vi "Scope1.vi"(2 "错误输入":errorcluster caption="错误输出") -> (0 "错误输出":errorcluster)   [LabVIEW 2018]
uses:
  <instrlib>/Tektronix DPO MSO 2000 4000 Series/Public/Configure/Configure Trigger (Edge).vi
  InOut/Reslut.vi
  <instrlib>/Tektronix DPO MSO 2000 4000 Series/Tektronix DPO MSO 2000 4000 Series.lvlib
panel:
  in  "结果输出":i32(listbox)
  in  "衰减挡位":T1 scale=1.0..4.0
  in  "触发电压":u64(ring)=200 items=["200mv"=200, "200mv"=0, "100mv"=100, "20mv"=20, "10mv"=10, "2mv"=2, "1mv"=1]
  in  "输入阻抗/Ω":u64(ring)=2 items=["1M", "75", "50"]
  out "时间波形":waveform(dbl)(graph)
  in  "电压范围":u64(ring)=10 items=["5v/dim"=5000000, "1v/dim"=1000000, "500mv/dim"=500000, "100mv/dim"=100000, "50mv/dim"=50000, "10mv/dim"=10000, "5mv/dim"=5000, "1mv/dim"=1000, "500uv/dim"=500, "100uv/dim"=100, "50uv/dim"=50, "10uv/dim"=10]
  in  "时间范围":u64(ring)=100000 items=["100ms/dim"=1000000000, "50ms/dim"=500000000, "10ms/dim"=100000000, "5ms/dim"=50000000, "1ms/dim"=10000000, "500us/dim"=5000000, "100us/dim"=1000000, "50us/dim"=500000, "10us/dim"=100000, "5us/dim"=50000, "1us/dim"=10000, "500ns/dim"=5000, "100ns/dim"=1000, "50ns/dim"=500, "10ns/dim"=100, "5ns/dim"=50, "1ns/dim"=10, "500ps/dim"=5, "100ps/dim"=1]
  in  "Channel":T2(ring)
  in  "测量状态":enum16{"设置参数", "等待", "采集", "结束", "调整衰减"}(ring)
  out "重频":string
  out "脉宽":string
  in  "结束测量":bool
  # "时间波形"
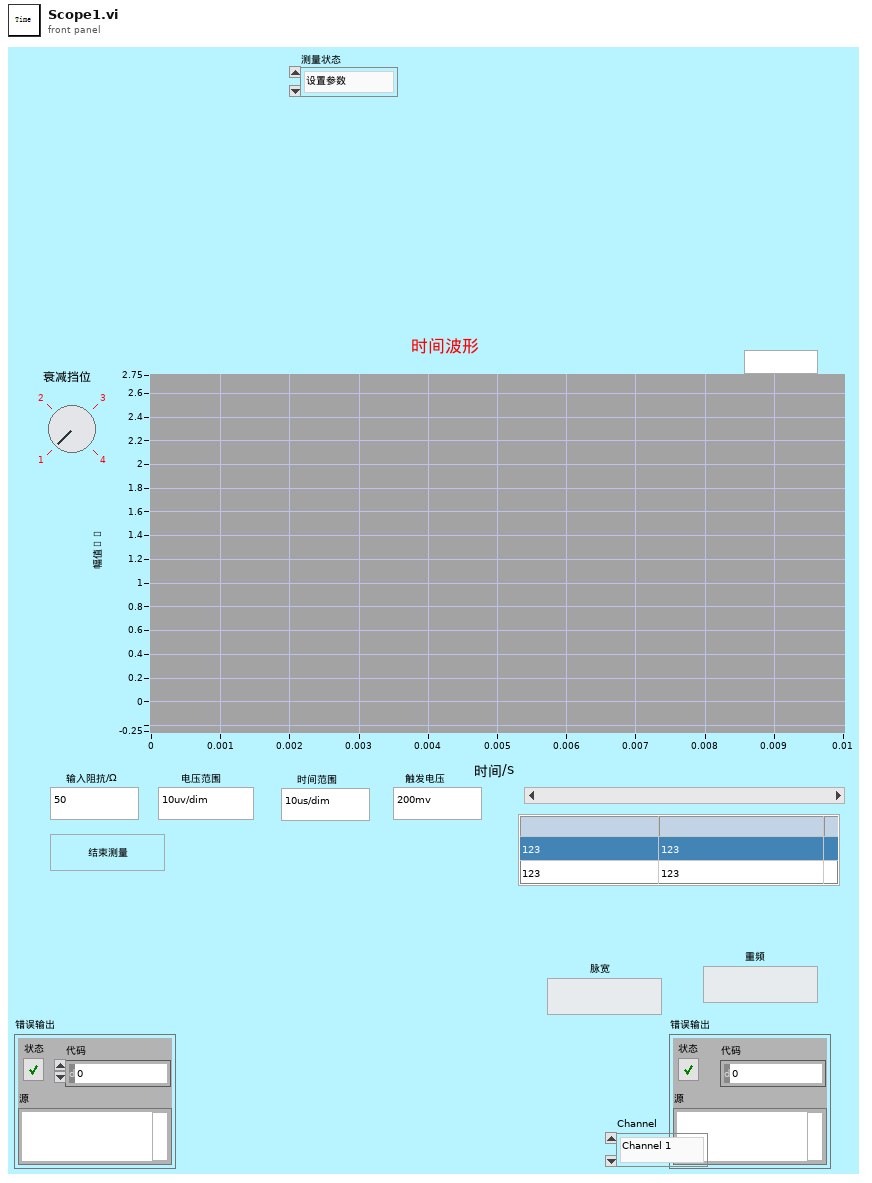
[diagram p1: front panel]
types:
  T1 = typedef "衰减片前面板.ctl" = u8
  T2 = enum16{"Channel 1", "Channel 2", "Channel 3", "Channel 4"}
  T3 = enum16{"光谱测量", "功率测量", "能量测量", "时间波形", "偏振测量", "近远场"}
  T4 = typedef "衰减片电机指令枚举器.ctl" = enum16{"归0", "停止", "运动", "轴设置", "通信连接", "读取位置"}
  T5 = typedef "衰减片电机枚举.ctl" = enum16{"小积分球衰减", "偏振仪衰减", "近场相机衰减", "远场相机衰减"}
  T6 = enum8{"Enabled", "Disabled", "Disabled and Grayed Out"}
  T7 = typedef "控制电机位置枚举器.ctl" = enum16{"远场扫描", "发散角扫描", "远场相机", "近场相机", "时间波形", "偏振", "能量", "功率", "光谱"}
  T8 = typedef "控制电机指令枚举器.ctl" = enum16{"归0", "停止", "运动", "轴设置", "通信连接"}
  T9 = typedef "控制电机枚举器.ctl" = enum16{"Z", "Y", "X", "发散角", "俯仰", "旋转"}
  T10 = enum16{"光谱测量", "功率测量", "能量测量", "时间波形测量", "偏振测量", "近远场测量"}
  T11 = typedef "衰减片电机位置枚举器.ctl" = enum16{"0倍", "10倍", "100倍", "1000倍"}
  T12 = cluster{"激光器型号":string, "X":dbl, "Y":dbl, "Z":dbl, "Rotate":dbl, "Pitching":dbl, "DivergeAngle":dbl, "衰减片位置":cluster{"小积分球位置":T11, "偏振仪位置 ":T11, "近场相机位置 ":T11, "远场相机位置":T11}, "Type":string, "Serial":string}
  T13 = typedef "IMAQ Image.ctl" = refnum<image>
  T14 = cluster{"示波器":cluster{"Channel (0:Channel 1)":enum16{"Channel 1", "Channel 2", "Channel 3", "Channel 4"}, "电压范围":dbl, "触发电压":dbl, "时间范围":dbl, " 示波器VISA":refnum<visa-resource-name>, "时间范围 标签":u64, "电压范围 标签":u64, "触发电压 标签":u64, "输入阻抗/Ω":u64, "示波器类型":bool}, "光谱仪":cluster{"SpecDataReference":refnum<queue>, "grating center":dbl, "Exposure Time (s)":dbl, "是否进行详细设置":bool, " 开始通信检查":bool, "通信成功？":bool, "波长":dbl, "LightField Automation out":refnum<class "LightField Automation.lvclass">}, " 近场相机":cluster{"曝光时间/us":dbl, "IP 地址":string, "ImageData":T13, " 曝光最大":i32, " 曝光最小":i32, "Camera Source":refnum<k21>, "近场X范围":dbl, "近场Y范围":dbl, "单个像元大小/um":dbl, "相机距离原点位置":dbl[], "是否测量发散角":bool, "光束类型(发散T)":bool, "聚焦透镜焦距mm":dbl}, " 偏振仪":cluster{"电压范围":u64, "触发电压":u64, "时间范围":u64, "波长范围":enum16{"可见光 400-700nm", "近红外 700-1100nm"}, "可见光偏振测量仪VISA":refnum<visa-resource-name>, "近红外偏振测量仪VISA":refnum<visa-resource-name>}, " 功率计":cluster{"通道":enum16{"Channel 1", "Channel 2"}, "工作波长":u32, "单位":u64, "时间范围":u64, "IP地址":string, "端口":u32, "是否需要散射片":bool}, "能量计":cluster{"通道":enum16{"Channel 1", "Channel 2"}, "工作波长":u32, "单位":u64, "时间范围":u64, "IP地址":string, "端口":u32, "能量计量程":enum16{"200uJ", "20uJ", "2uJ", "200nJ"}}, "电机":cluster{"Channel (0:Channel 1)":enum16{"Channel 1", "Channel 2", "Channel 3", "Channel 4"}, "电压范围":u64, "触发电压":u64, "时间范围":u64}, " 远场相机":cluster{"曝光时间/us":i32, "IP 地址":string, "ImageData":T13, "  增益最大":i32, "  增益最小":i32, " 曝光最大":i32, " 曝光最小":i32, "ImageData B":T13, "是否远场测量":bool}}
  T15 = cluster{"Channel (0:Channel 1)":enum16{"Channel 1", "Channel 2", "Channel 3", "Channel 4"}, "电压范围":dbl, "触发电压":dbl, "时间范围":dbl, " 示波器VISA":refnum<visa-resource-name>, "时间范围 标签":u64, "电压范围 标签":u64, "触发电压 标签":u64, "输入阻抗/Ω":u64, "示波器类型":bool}
  T16 = cluster{"波形":waveform(dbl), "脉宽":string, "重频":string, "脉冲宽度Uint":string, "重复频率Uint":string}
  T17 = cluster{"任务":cluster{"功率任务":bool, "能量任务":bool, "时间波形任务":bool, "光谱任务":bool, "偏振任务":bool, "近远场任务":bool}, "通信":cluster{"功率通信":bool, "能量通信":bool, "时间波形通信":bool, "光谱通信":bool, "偏振通信":bool, "近远场通信":bool}}
  T18 = cluster{"功率通信":bool, "能量通信":bool, "时间波形通信":bool, "光谱通信":bool, "偏振通信":bool, "近远场通信":bool}
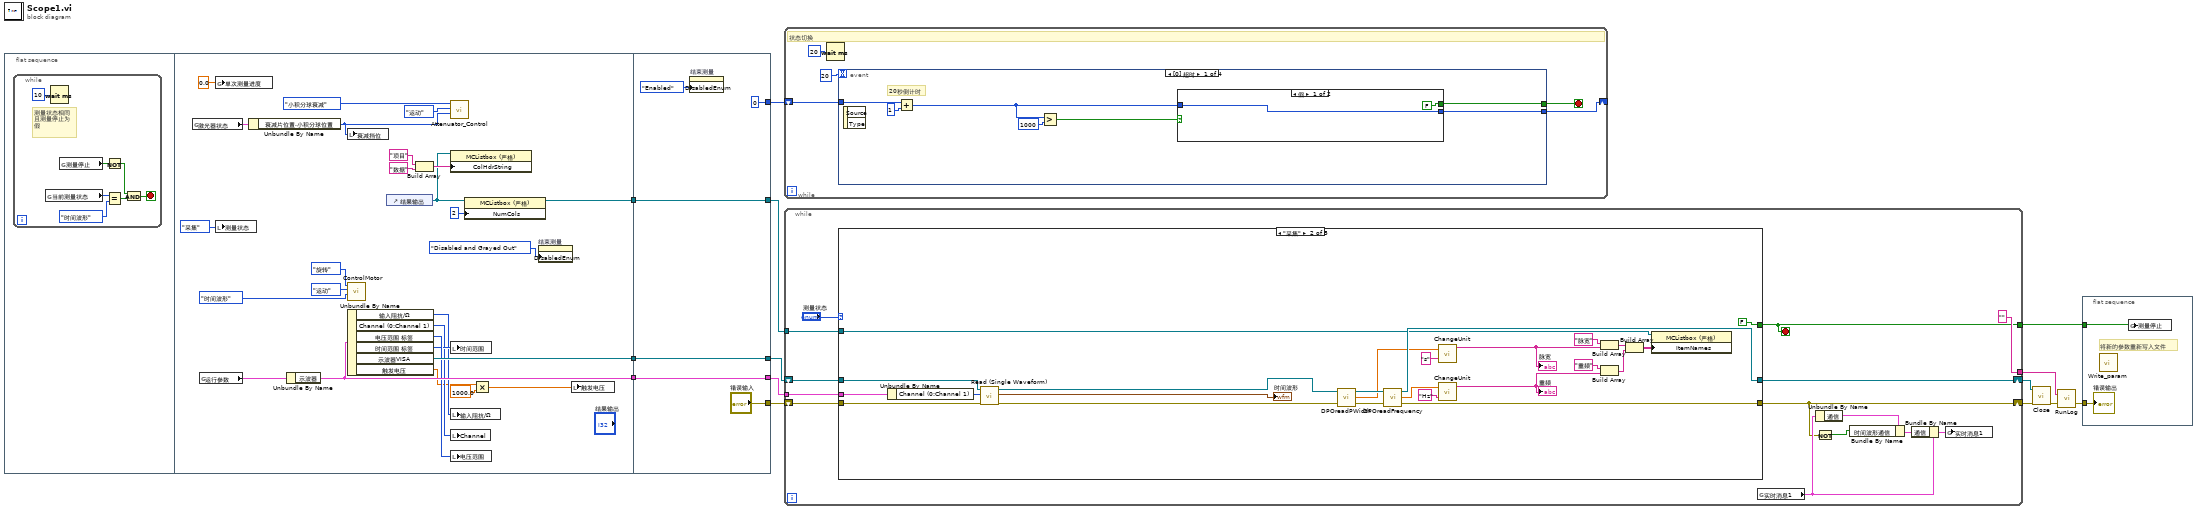
[diagram p0: block diagram]
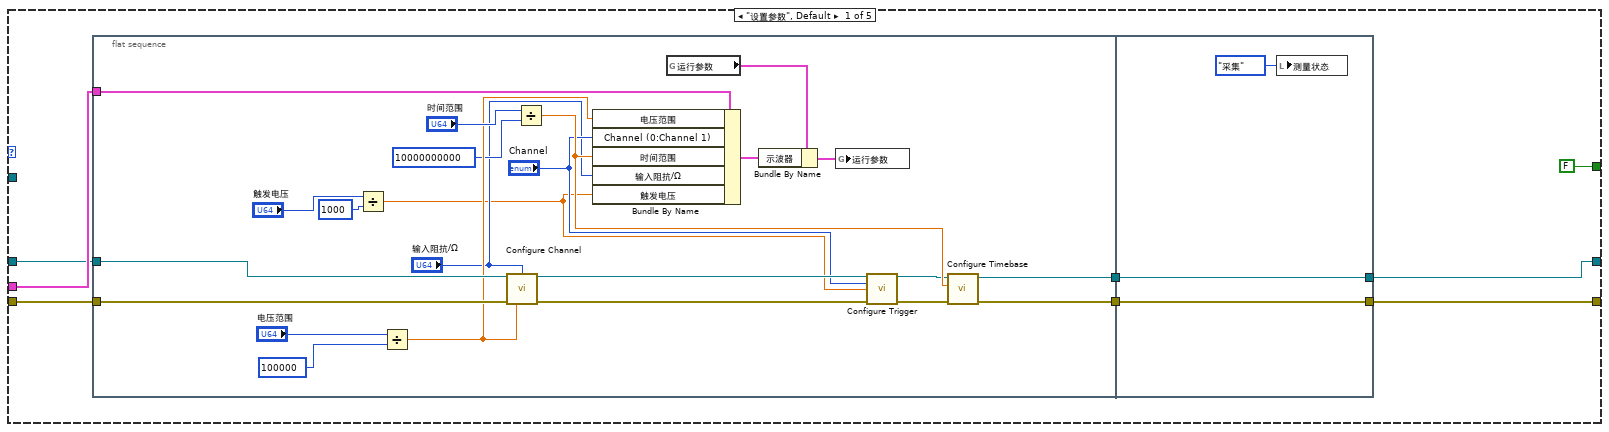
[diagram p2: hidden frame]
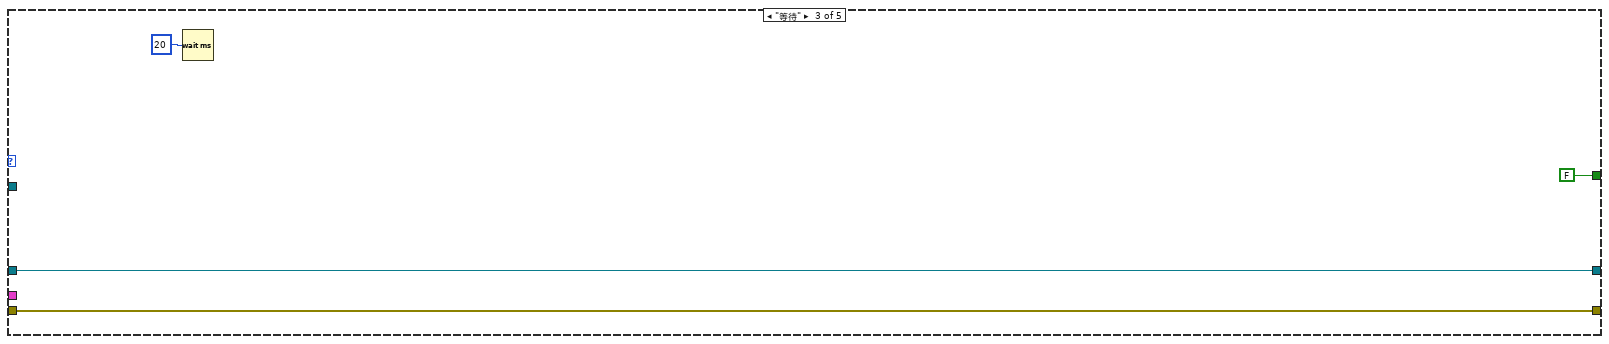
[diagram p3: hidden frame]
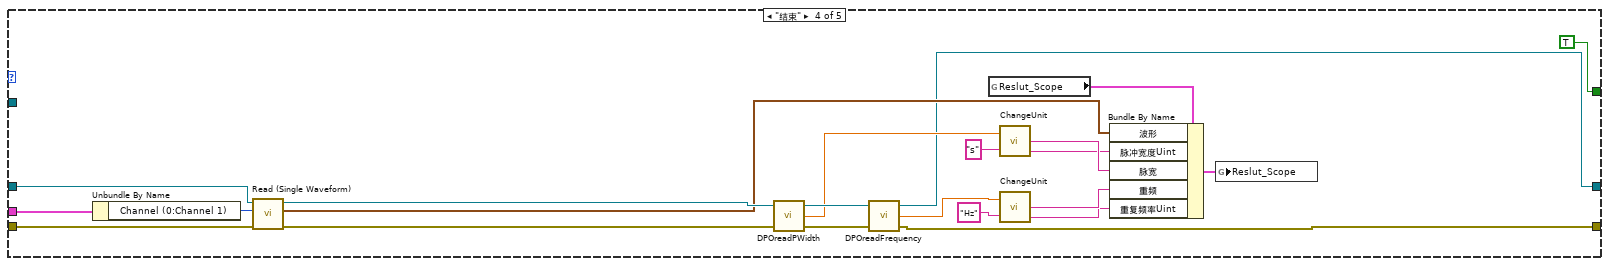
[diagram p4: hidden frame]
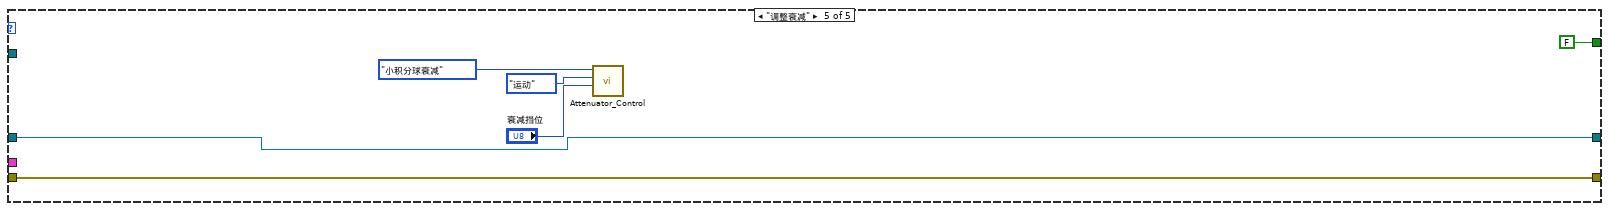
[diagram p5: hidden frame]
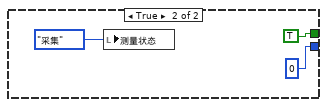
[diagram p6: hidden frame]
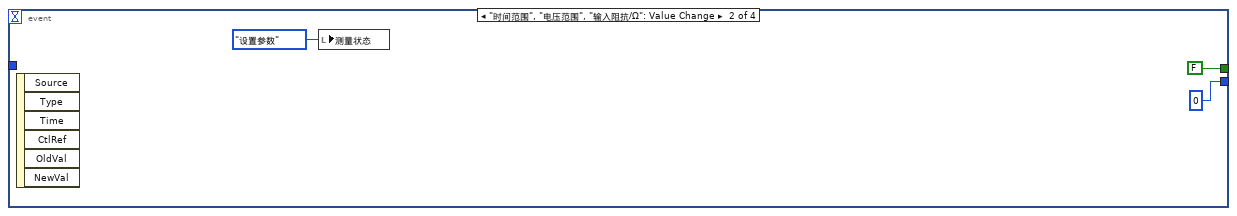
[diagram p7: hidden frame]
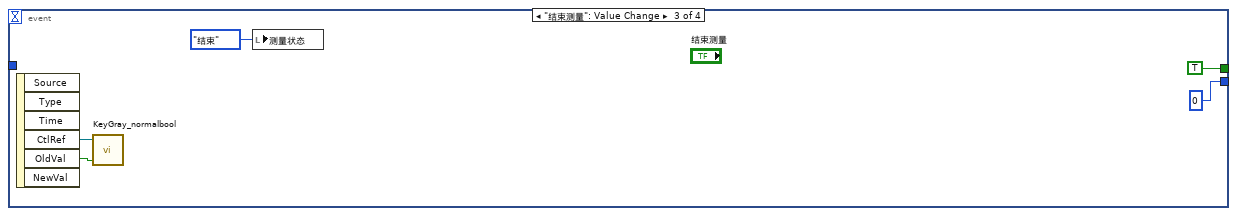
[diagram p8: hidden frame]
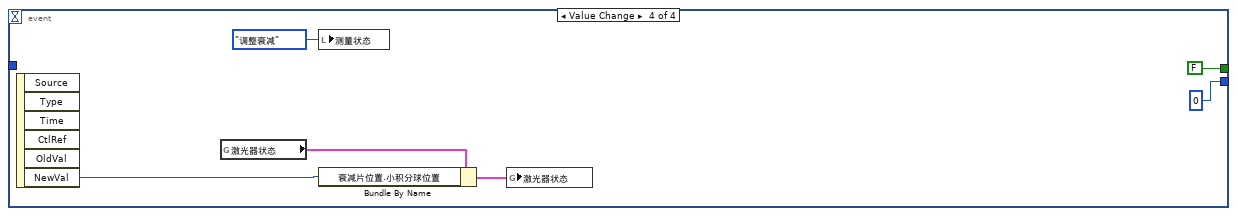
[diagram p9: hidden frame]
diagram:
  n1 = flat-sequence {
    tunnel: [w47] -> w6
    tunnel: [w45] -> w5
    tunnel: [w22] -> w2
    tunnel: [w52] -> w13
    tunnel: [w53] -> w14
    tunnel: w6 -> [w53]
    tunnel: w5 -> [w52]
    tunnel: [0] -> w7
    tunnel: [w49] -> w3
    tunnel: w2 -> [w49]
    tunnel: ["错误输入"] -> w1
    frame #0 {
      n2 = while {
        stop <- w19 stop-if-true
        # "测量状态相同\n且测量停止为\n假"
        n3 = global read "参数.vi" "当前测量状态"() -> (w21:T10)
        n4 = Wait (ms)(milliseconds to wait=u32 10 ("等待时间（毫秒）")) -> ()  [unwired: 1 out]
        n5 = global read "参数.vi" "测量停止"() -> (w17:bool)
        n6 = Not(x=w17) -> (.not. x?=w18:bool)
        n7 = Equal?(x=w21, y=T3."时间波形" ("当前测量状态")) -> (x = y?=w16:bool)
        n8 = And(x=w18, y=w16) -> (x .and. y?=w19:bool)
      }
    }
    frame #1 {
      n9 = global read "参数.vi" "激光器状态"() -> (w35:T12)
      n10 = global read "参数.vi" "运行参数"() -> (w46:T14)
      n11 = global write "globalMessage.vi" "单次测量进度"(0.0 ("单次测量进度")) -> ()
      n12 = local write "测量状态"(enum16{"设置参数", "等待", "采集"}."采集" ("测量状态")) -> ()
      n13 = Unbundle By Name(w35) -> ("衰减片位置.小积分球位置"=w28:T11)
      n14 = Unbundle By Name(w46) -> ("示波器"=w45:T15)
      n15 = local write "衰减挡位"(w28) -> ()
      n16 = call "ControlMotor.vi"("控制电机"=控制电机枚举器."旋转", "控制电机指令"=控制电机指令枚举器."运动", "位置"=控制电机位置枚举器."时间波形") -> ()  [unwired: 5 in, 1 out]
      n17 = Unbundle By Name(w45) -> ("输入阻抗/Ω"=w40:u64, "Channel (0:Channel 1)"=w41:T2, "电压范围 标签"=w44:u64, "时间范围 标签"=w43:u64, "示波器VISA"=w47:refnum<visa-resource-name>, "触发电压"=w39:dbl)
      n18 = control-ref of="结果输出"() -> (w23:refnum<vi>)
      n19 = Build Array("项目", "数据") -> (w24:string[])
      n20 = call "Attenuator_Control.vi"("位置"=w28, "控制电机指令"=衰减片电机指令枚举器."运动", "电机"=衰减片电机枚举."小积分球衰减") -> ()  [unwired: 2 in, 2 out]
      n21 = property on="属性节点" class="MCListbox (严格)"(reference=w23, "ColHdrString"=w24) -> ()  [unwired: 1 in, 2 out]
      n22 = local write "时间范围"(w43) -> ()
      n23 = local write "输入阻抗/Ω"(w40) -> ()
      n24 = local write "Channel"(w41) -> ()
      n25 = local write "电压范围"(w44) -> ()
      n26 = property on="属性节点" class="MCListbox (严格)"(reference=w23, "NumCols"=u32 2 ("列数")) -> (reference out=w22:refnum<vi>)  [unwired: 1 in, 1 out]
      n27 = Multiply(x=w39, y=1000.0) -> (x*y=w37:dbl)
      n28 = property on="结束测量" class="Bool (严格)"("DisabledEnum"=T6."Disabled and Grayed Out" ("禁用")) -> ()  [unwired: 2 in, 2 out]
      n29 = local write "触发电压"(w37) -> ()
    }
    frame #2 {
      n30 = property on="结束测量" class="Bool (严格)"("DisabledEnum"=T6."Enabled" ("禁用")) -> ()  [unwired: 2 in, 2 out]
    }
  }
  n31 = while "While循环" {
    shift-right: [w54] -> _
    shift-left: w7 -> [w55]
    stop <- w57 stop-if-true
    # "状态切换"
    n32 = Wait (ms)(milliseconds to wait=u32 20 ("等待时间（毫秒）")) -> ()  [unwired: 1 out]
    n33 = event shown="[0] 超时" {
      selector: _ -> [_ _ _ _]
      dyn-events: _ -> [_ _ _ _]
      timeout: 20 -> [_ _ _ _]
      tunnel: [w60 FALSE TRUE FALSE] -> w57
      tunnel: w55 -> [w65 _ _ _]
      tunnel: [w61 0 0 0] -> w54
      event Timeout {
        # "20秒倒计时"
        n34 = event-data() -> ()  [unwired: 1 in, 2 out]
        n35 = Add(x=w65, y=1) -> (x+y=w59:i32)
        n36 = Greater?(x=w59, y=1000) -> (0:w62:bool)
        n37 = case shown="假" w62 {
          tunnel: [w67 0] -> w61
          tunnel: [FALSE TRUE] -> w60
          tunnel: w59 -> [w67 _]
          frame False {
          }
          frame True {
            n38 = local write "测量状态"(enum16{"设置参数", "等待", "采集", "结束"}."采集" ("测量状态")) -> ()
          }
        }
      }
      event "时间范围", "电压范围", "输入阻抗/Ω": Value Change {
        n39 = event-data() -> ()  [unwired: 1 in, 6 out]
        n40 = local write "测量状态"(enum16{"设置参数", "等待", "采集", "结束"}."设置参数" ("测量状态")) -> ()
      }
      event "结束测量": Value Change {
        n41 = event-data() -> ("CtlRef"=w78:refnum<vi>, "OldVal"=w77:bool)  [unwired: 1 in, 4 out]
        n42 = call "KeyGray_normalbool.vi"("OldVal"=w77, "引用"=w78) -> ()  [unwired: 2 in]
        n43 = local write "测量状态"(enum16{"设置参数", "等待", "采集", "结束"}."结束" ("测量状态")) -> ()
      }
      event Value Change {
        n44 = event-data() -> ("NewVal"=w81:T1)  [unwired: 1 in, 5 out]
        n45 = global read "参数.vi" "激光器状态"() -> (w82:T12)
        n46 = local write "测量状态"(enum16{"设置参数", "等待", "采集", "结束", "调整衰减"}."调整衰减" ("测量状态")) -> ()
        n47 = Bundle By Name(cluster=w82, "衰减片位置.小积分球位置"=w81) -> (w80:T12)
        n48 = global write "参数.vi" "激光器状态"(w80) -> ()
      }
    }
  }
  n49 = while {
    shift-right: [w98] -> w11
    shift-left: w14 -> [w97]
    shift-right: [w87] -> w12
    shift-left: w1 -> [w86]
    tunnel: w13 -> [w96]
    tunnel: ["" ("source")] -> w9
    tunnel: [w88] -> w4
    tunnel: w3 -> [w85]
    stop <- w88 stop-if-true
    n50 = case shown="\"采集\"" "测量状态" {
      tunnel: w97 -> [w105 w144 w160 w170 w188]
      tunnel: [w102 w156 w160 w163 w188] -> w98
      tunnel: [w103 w155 w159 w162 w187] -> w87
      tunnel: w86 -> [w104 w143 w159 w169 w187]
      tunnel: w96 -> [w106 w154 _ w171 _]
      tunnel: [FALSE FALSE FALSE TRUE FALSE] -> w88
      tunnel: w85 -> [_ w140 _ _ _]
      frame "设置参数", Default {
        n51 = flat-sequence {
          tunnel: w106 -> [w129]
          tunnel: w105 -> [w128]
          tunnel: w104 -> [w127]
          tunnel: [w126] -> w101
          tunnel: [w125] -> w100
          tunnel: [w131] -> w102
          tunnel: [w132] -> w103
          tunnel: w101 -> [w132]
          tunnel: w100 -> [w131]
          frame #0 {
            n52 = Divide(x="触发电压", y=u64 1000) -> (x/y=w108:dbl)
            n53 = Divide(x="电压范围", y=u64 100000) -> (x/y=w121:dbl)
            n54 = call <instrlib>:"Configure Channel.vi"("VISA resource name"=w128, "Input Impedance (0: 1M ohm)"="输入阻抗/Ω", "error in (no error)"=w127, "Vertical Range (10.0 V)"=w121) -> ("VISA resource name out"=w115:refnum<visa-resource-name>, "error out"=w113:errorcluster)  [unwired: 10 in]
            n55 = Divide(x="时间范围", y=u64 10000000000) -> (x/y=w120:dbl)
            n56 = Bundle By Name(cluster=w129, "电压范围"=w121, "Channel (0:Channel 1)"="Channel", "时间范围"=w120, "输入阻抗/Ω"="输入阻抗/Ω", "触发电压"=w108) -> (w117:T15)
            n57 = global read "参数.vi" "运行参数"() -> (w119:T14)
            n58 = Bundle By Name(cluster=w119, "示波器"=w117) -> (w118:T14)
            n59 = global write "参数.vi" "运行参数"(w118) -> ()
            n60 = call-poly <instrlib>:"Configure Trigger.vi"("VISA resource name"=w115, "Trigger Source (0: Channel 1)"="Channel", "Trigger Level (0.0 V)"=w108, "error in (no error)"=w113) -> ("VISA resource name out"=w114:refnum<visa-resource-name>, "error out"=w112:errorcluster)  [unwired: 10 in]
            n61 = call <instrlib>:"Configure Timebase.vi"("error in (no error)"=w112, "Timebase (0.0005 s)"=w120, "VISA resource name"=w114) -> ("error out"=w126:errorcluster, "VISA resource name out"=w125:refnum<visa-resource-name>)  [unwired: 7 in]
          }
          frame #1 {
            n62 = local write "测量状态"(enum16{"设置参数", "等待", "采集", "结束"}."采集" ("测量状态")) -> ()
          }
        }
      }
      frame "采集" {
        n63 = Unbundle By Name(w154) -> ("Channel (0:Channel 1)"=w153:T2)
        n64 = call <instrlib>:"Read (Single Waveform).vi"("error in (no error)"=w143, "Channel (0: Channel 1)"=w153, "VISA resource name"=w144) -> ("error out"=w141:errorcluster, "Waveform Graph"=→"时间波形":waveform(dbl), "VISA resource name out"=w142:refnum<visa-resource-name>)  [unwired: 6 in]
        n65 = call "DPOreadPWidth.vi"("错误输入（无错误）"=w141, "VISA资源名称"=w142) -> ("错误输出"=w151:errorcluster, "上升沿时间"=w150:dbl, "VISA资源名称输出"=w152:refnum<visa-resource-name>)  [unwired: 1 in]
        n66 = call "DPOreadFrequency.vi"("错误输入（无错误）"=w151, "VISA资源名称"=w152) -> ("错误输出"=w155:errorcluster, "重复频率"=w148:dbl, "VISA资源名称输出"=w156:refnum<visa-resource-name>)  [unwired: 1 in]
        n67 = call "ChangeUnit.vi"("change in"=w150, "unit in"="s") -> ("change out"=w138:string)  [unwired: 2 out]
        "脉宽" <- w138
        n68 = call "ChangeUnit.vi"("change in"=w148, "unit in"="Hz") -> ("change out"=w135:string)  [unwired: 2 out]
        "重频" <- w135
        n69 = Build Array("脉宽" ("字符串"), w138) -> (w137:string[])
        n70 = Build Array("重频" ("字符串"), w135) -> (w134:string[])
        n71 = Build Array(w137, w134) -> (w133:string[][])
        n72 = property on="属性节点" class="MCListbox (严格)"(reference=w140, "ItemNames"=w133) -> ()  [unwired: 1 in, 2 out]
      }
      frame "等待" {
        n73 = Wait (ms)(milliseconds to wait=u32 20 ("等待时间（毫秒）")) -> ()  [unwired: 1 out]
      }
      frame "结束" {
        n74 = Unbundle By Name(w171) -> ("Channel (0:Channel 1)"=w180:T2)
        n75 = call <instrlib>:"Read (Single Waveform).vi"("error in (no error)"=w169, "Channel (0: Channel 1)"=w180, "VISA resource name"=w170) -> ("error out"=w172:errorcluster, "Waveform Graph"=w168:waveform(dbl), "VISA resource name out"=w179:refnum<visa-resource-name>)  [unwired: 6 in]
        n76 = call "DPOreadPWidth.vi"("错误输入（无错误）"=w172, "VISA资源名称"=w179) -> ("错误输出"=w177:errorcluster, "上升沿时间"=w176:dbl, "VISA资源名称输出"=w178:refnum<visa-resource-name>)  [unwired: 1 in]
        n77 = call "DPOreadFrequency.vi"("错误输入（无错误）"=w177, "VISA资源名称"=w178) -> ("错误输出"=w162:errorcluster, "重复频率"=w174:dbl, "VISA资源名称输出"=w163:refnum<visa-resource-name>)  [unwired: 1 in]
        n78 = global read "Reslut.vi" "Reslut_Scope"() -> (w161:T16)
        n79 = call "ChangeUnit.vi"("change in"=w176, "unit in"="s") -> ("DataOut"=w167:string, "UintOut"=w166:string)  [unwired: 1 out]
        n80 = call "ChangeUnit.vi"("change in"=w174, "unit in"="Hz") -> ("DataOut"=w165:string, "UintOut"=w164:string)  [unwired: 1 out]
        n81 = Bundle By Name(cluster=w161, "波形"=w168, "脉冲宽度Uint"=w166, "脉宽"=w167, "重频"=w165, "重复频率Uint"=w164) -> (w181:T16)
        n82 = global write "Reslut.vi" "Reslut_Scope"(w181) -> ()
      }
      frame "调整衰减" {
        n83 = call "Attenuator_Control.vi"("位置"="衰减挡位", "控制电机指令"=衰减片电机指令枚举器."运动", "电机"=衰减片电机枚举."小积分球衰减") -> ()  [unwired: 2 in, 2 out]
      }
    }
    n84 = global read "globalMessage.vi" "实时消息1"() -> (w93:T17)
    n85 = Unbundle By Name(w93) -> ("通信"=w94:T18)
    n86 = Not(x=w87) -> (.not. x?=w90:bool)
    n87 = Bundle By Name(cluster=w94, "时间波形通信"=w90) -> (w92:T18)
    n88 = Bundle By Name(cluster=w93, "通信"=w92) -> (w91:T17)
    n89 = global write "globalMessage.vi" "实时消息1"(w91) -> ()
  }
  n90 = call <instrlib>:"Close.vi"("error in (no error)"=w12, "VISA resource name"=w11) -> ("error out"=w10:errorcluster)  [unwired: 9 in]
  n91 = call "RunLog.vi"("error in"=w10, "Message"=w9) -> ("error out"=w8:errorcluster)  [unwired: 1 in]
  n92 = flat-sequence {
    tunnel: w8 -> [w190]
    tunnel: w4 -> [w189]
    frame #0 {
      # "将新的参数重新写入文件"
      n93 = call "Write_param.vi"() -> ()  [unwired: 12 in]
      n94 = global write "参数.vi" "测量停止"(w189) -> ()
      "错误输出" <- w190
    }
  }
